vi "Write Cell.vi"(8 "error in":errorcluster, 10 "Cell":u8, 11 "PAS Cell Data in":refnum<class "PAS Cell Data.lvclass">=refnum) -> (0 "error out":errorcluster, 3 "PAS Cell Data out":refnum<class "PAS Cell Data.lvclass">)   [LabVIEW 2014, in "PAS Cell Data.lvclass"]
uses:
  PAS Cell Data.lvclass
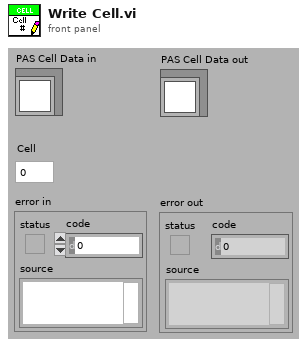
[diagram p1: front panel]
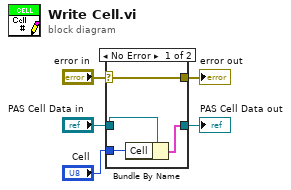
[diagram p0: block diagram]
diagram:
  n1 = case shown="No Error" "error in" {
    selector: "error in" -> [w9 w10]
    tunnel: [w9 w10] -> w4
    tunnel: [w7 w11] -> w2
    tunnel: "PAS Cell Data in" -> [w8 w11]
    tunnel: "Cell" -> [w6 _]
    frame No Error {
      n2 = Bundle By Name(cluster=w8, "Cell"=w6) -> (w7:cluster{})
    }
    frame Error {
    }
  }
  "error out" <- w4
  "PAS Cell Data out" <- w2
